vi "Shooter Wheel Set.vi"(7 "RPM":dbl format="%#_13g", 8 "CounterDevRef in":T9={"DevStatus"={"status"=FALSE, "code"=0, "source"=""}, "CntIndex"=enum."Invalid"}, 9 "MotorControlDevRef":T2={"DeviceStatus"={"status"=FALSE, "code"=0, "source"=""}, "Type"=enum."PWM", "PWM"={"PWM Channel"=enum."Invalid", "DeadBand"={"Name"="", "maxPositivePwm"=0, "minPositivePwm"=0, "centerPwm"=0, "maxNegativePwm"=0, "minNegativePwm"=0, "angularRange"=0}}, "CAN"={"Device Number"=0, "Control Mode"=enum."Percent VBus", "Semaphore"=refnum, "Max Vout"=12.0, "TalonSRX Control Mode"=enum."Percent VBus"}, "Invert"=FALSE}, 10 "DevRef":string, 11 "data value":T1={"Period (ms)"=20, "TBH Gain"=0.5, "Priority"=100}) -> (0 "Error Out":errorcluster, 3 "Shooter Wheel DevRef Out":T11={"Shooter Config reference"=refnum, "Shooter Data"={"MotorControlDevRef"={"DeviceStatus"={"status"=FALSE, "code"=0, "source"=""}, "Type"=enum."PWM", "PWM"={"PWM Channel"=enum."Invalid", "DeadBand"={"Name"="", "maxPositivePwm"=0, "minPositivePwm"=0, "centerPwm"=0, "maxNegativePwm"=0, "minNegativePwm"=0, "angularRange"=0}}, "CAN"={"Device Number"=0, "Control Mode"=enum."Percent VBus", "Semaphore"=refnum, "Max Vout"=12.0, "TalonSRX Control Mode"=enum."Percent VBus"}, "Invert"=FALSE}, "CounterDevRef in"={"DevStatus"={"status"=FALSE, "code"=0, "source"=""}, "CntIndex"=enum."Ctr 0"}, "RPM Desired"=refnum, "RPM Actual"=refnum}})   [LabVIEW 2015, in "Shooter _Wheel.lvlib"]
doc: "Help By FRC Team 836 - The RoboBees\n\nThis VI sets the operating parameters of a shooter wheel."
uses:
  <userlib>/836-Library/Motion_Control/Shooter_Wheel/Shooter _Wheel.lvlib
  <userlib>/836-Library/Motion_Control/Shooter_Wheel/ShooterControl.ctl
  <userlib>/836-Library/Motion_Control/Shooter_Wheel/ShooterConfig.ctl
  <userlib>/836-Library/Motion_Control/Shooter_Wheel/ShooterData.ctl
  <vilib>/Rock Robotics/WPI/MotorControl/WPI_MotorControlDeviceRef.ctl
  <vilib>/Rock Robotics/WPI/MotorControl/WPI_MotorControlType.ctl
  <vilib>/Rock Robotics/SystemInterfaces/DIO/FPGA_DIOPWMChannel.ctl
  <vilib>/Rock Robotics/WPI/PWM/WPI_PWMDeadband.ctl
  <vilib>/Rock Robotics/WPI/CAN/Jaguar/SubVIs/WPI_CANJaguar_ControlMode.ctl
  <vilib>/Rock Robotics/WPI/CAN/TalonSRX/WPI_CANTalonSRX_APIControlMode.ctl
  <vilib>/Rock Robotics/WPI/Counter/WPI_CounterDevRef.ctl
  <vilib>/Rock Robotics/SystemInterfaces/Counter/FPGA_CounterCtrSystemIndex.ctl
  <userlib>/836-Library/Motion_Control/Shooter_Wheel/Shooter Wheel.lvlib
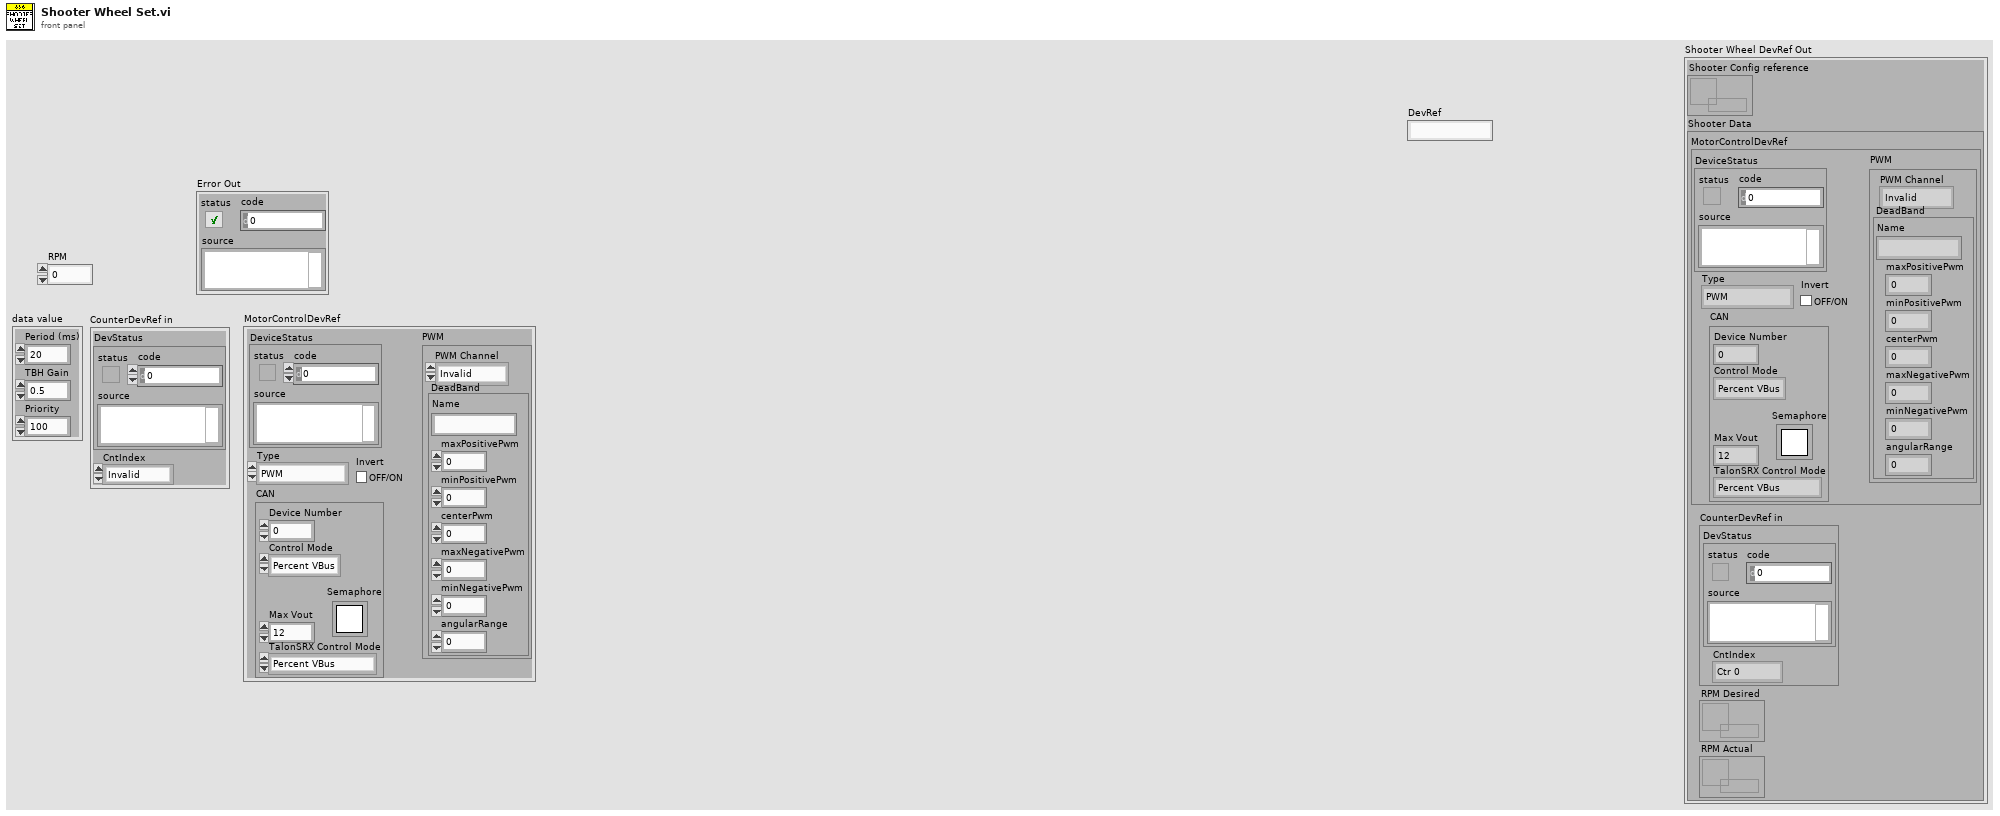
[diagram p1: front panel]
types:
  T1 = typedef "Shooter Wheel.lvlib/ShooterConfig.ctl" = cluster{"Period (ms)":i64, "TBH Gain":dbl, "Priority":i32}
  T2 = typedef "WPI_MotorControlDeviceRef.ctl" = cluster{"DeviceStatus":errorcluster, "Type":T3, "PWM":cluster{"PWM Channel":T4, "DeadBand":T5}, "CAN":cluster{"Device Number":u8, "Control Mode":T6, "Semaphore":T7, "Max Vout":dbl, "TalonSRX Control Mode":T8}, "Invert":bool}
  T3 = typedef "WPI_MotorControlType.ctl" = enum16{"PWM", "CAN", "CANTalonSRX"}
  T4 = typedef "FPGA_DIOPWMChannel.ctl" = enum8{"PWM 0", "PWM 1", "PWM 2", "PWM 3", "PWM 4", "PWM 5", "PWM 6", "PWM 7", "PWM 8", "PWM 9", "PWM MXP 0", "PWM MXP 1", "PWM MXP 2", "PWM MXP 3", "PWM MXP 4", "PWM MXP 5", "PWM MXP 6", "PWM MXP 7", "PWM MXP 8", "PWM MXP 9", "Invalid"}
  T5 = typedef "WPI_PWMDeadband.ctl" = cluster{"Name":string, "maxPositivePwm":i32, "minPositivePwm":i32, "centerPwm":i32, "maxNegativePwm":i32, "minNegativePwm":i32, "angularRange":u16}
  T6 = typedef "WPI_CANJaguar_ControlMode.ctl" = enum8{"Percent VBus", "Current", "Speed", "Position", "Voltage"}
  T7 = typedef "Semaphore RefNum" = refnum<k1>
  T8 = typedef "WPI_CANTalonSRX_APIControlMode.ctl" = enum8{"Percent VBus", "Speed", "Position", "Slave", "Unchanged / Invalid", "Voltage Compensation", "Current", "Motion Profile"}
  T9 = typedef "WPI_CounterDevRef.ctl" = cluster{"DevStatus":errorcluster, "CntIndex":T10}
  T10 = typedef "FPGA_CounterCtrSystemIndex.ctl" = enum8{"Ctr 0", "Ctr 1", "Ctr 2", "Ctr 3", "Ctr 4", "Ctr 5", "Ctr 6", "Ctr 7", "Invalid"}
  T11 = typedef "Shooter Wheel.lvlib/ShooterControl.ctl" = cluster{"Shooter Config reference":refnum<data-value>, "Shooter Data":T12}
  T12 = typedef "Shooter Wheel.lvlib/ShooterData.ctl" = cluster{"MotorControlDevRef":T2, "CounterDevRef in":T9, "RPM Desired":refnum<k33>, "RPM Actual":refnum<k33>}
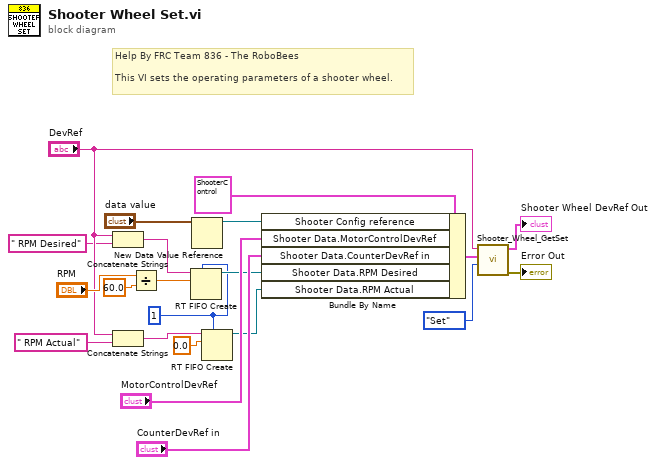
[diagram p0: block diagram]
diagram:
  w6 = u32 1 ("size (10)")
  # "Help By FRC Team 836 - The RoboBees\n\nThis VI sets the operating parameters of a shooter wheel."
  n1 = Concatenate Strings("DevRef", " RPM Desired" ("string")) -> (w7:string)
  n2 = Concatenate Strings("DevRef", " RPM Actual" ("string")) -> (w5:string)
  n3 = Divide(x="RPM", y=60.0) -> (x/y=w2:dbl)
  n4 = RT FIFO Create(0:w7, 1:w2, 4:w6) -> (8:w9:refnum<k33>)  [unwired: 5 in, 2 out]
  n5 = New Data Value Reference(data value="data value") -> (data value reference=w8:refnum<data-value>)  [unwired: 1 in, 1 out]
  n6 = RT FIFO Create(0:w5, 1:0.0, 4:w6) -> (8:w10:refnum<k33>)  [unwired: 5 in, 2 out]
  n7 = Bundle By Name(cluster=T11 {"Shooter Config reference"=refnum, "Shooter Data"={"MotorControlDevRef"={"DeviceStatus"={"status"=FALSE, "code"=0, "source"=""}, "Type"=enum."PWM", "PWM"={"PWM Channel"=enum."Invalid", "DeadBand"={"Name"="", "maxPositivePwm"=0, "minPositivePwm"=0, "centerPwm"=0, "maxNegativePwm"=0, "minNegativePwm"=0, "angularRange"=0}}, "CAN"={"Device Number"=0, "Control Mode"=enum."Percent VBus", "Semaphore"=refnum, "Max Vout"=12.0, "TalonSRX Control Mode"=enum."Percent VBus"}, "Invert"=FALSE}, "CounterDevRef in"={"DevStatus"={"status"=FALSE, "code"=0, "source"=""}, "CntIndex"=enum."Ctr 0"}, "RPM Desired"=refnum, "RPM Actual"=refnum}}, "Shooter Config reference"=w8, "Shooter Data.MotorControlDevRef"="MotorControlDevRef", "Shooter Data.CounterDevRef in"="CounterDevRef in", "Shooter Data.RPM Desired"=w9, "Shooter Data.RPM Actual"=w10) -> (w15:T11)
  n8 = call <userlib>:"Shooter_Wheel_GetSet.vi"("Enum"=enum16{"Set", "Get"}."Set", "Shooter Wheel DevRef In"=w15, "DevRef"="DevRef") -> ("Error Out"=→"Error Out":errorcluster, "Shooter Wheel DevRef Out"=→"Shooter Wheel DevRef Out":T11)  [unwired: 7 in]
